vi "FlatToRichw4lvgrpc_Msg_ToClient_2.vi"(5 "OutputClusterType":T1, 11 "InputCluster":T2) -> (3 "OutputCluster":T1)   [LabVIEW 2019, in "Generated_server.lvlib"]
uses:
  Generated_server.lvlib
  w4lvgrpc_Msg_ToClient_2.ctl
  w4lvgrpc_Msg_ToClient_2_Flat.ctl
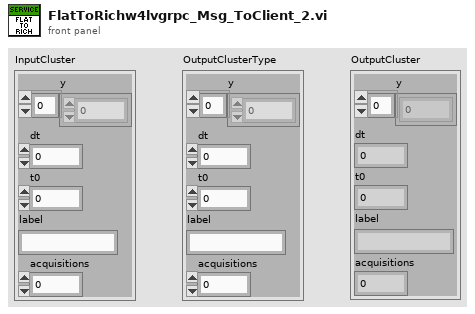
[diagram p1: front panel]
types:
  T1 = typedef "Generated_server.lvlib/w4lvgrpc_Msg_ToClient_2.ctl" = cluster{"y":dbl[], "dt":dbl, "t0":dbl, "label":string, "acquisitions":i32}
  T2 = typedef "Generated_server.lvlib/w4lvgrpc_Msg_ToClient_2_Flat.ctl" = cluster{"y":dbl[], "dt":dbl, "t0":dbl, "label":string, "acquisitions":i32}
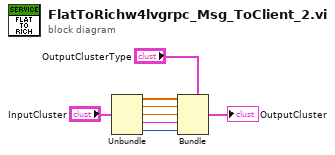
[diagram p0: block diagram]
diagram:
  n1 = Unbundle "Unbundle"("InputCluster") -> ("y"=w5:dbl[], "dt"=w4:dbl, "t0"=w3:dbl, "label"=w2:string, "acquisitions"=w1:i32)
  n2 = Bundle "Bundle"(cluster="OutputClusterType", "y"=w5, "dt"=w4, "t0"=w3, "label"=w2, "acquisitions"=w1) -> (→"OutputCluster":T1)
